vi "IRR-check-timeframe.vi"(8 "error in":errorcluster, 10 "Clk":dbl, 11 "ProcName":string) -> (0 "error out":errorcluster, 1 "ENG.CALL":cluster{"CMD":T1, "data":variant}, 2 "Report":string, 5 "Will Irrigate?":bool)   [LabVIEW 2024]
uses:
  controls/state-engine.ctl
  controls/type.eng-call.proc-insert.ctl
  controls/UiStepBuilder.ctl
  controls/type.step-builder.ctl
  io.interface.serial.vi
  build.flowToVarient.vi
  <vilib>/Utility/error.llb/Clear Errors.vi
  Polymorphics/variantCtrl.polymorphic.vi
  Polymorphics/variantCtrlStepFunction.vi
  Polymorphics/variantCtrlSetpoint.vi
  Polymorphics/variantCtrlString.vi
  proc.util.enumToStrStepVar.vi
  util.DelimitedStringFromArray.vi
  Polymorphics/variantCtrlNumber.vi
  util.DelimitedStringToArray.vi
  proc.util.validateParamExist.vi
  <vilib>/Utility/error.llb/Trim Whitespace.vi
  <vilib>/Utility/error.llb/Trim Whitespace One-Sided.vi
  globals/globals-engine.vi
  Polymorphics/variantCtrlIo.vi
  util.environment.vi
  util-address-parser.vi
  util-address-builder.vi
  util.DO.ToString.vi
  Polymorphics/io.command-builder.vi
  Polymorphics/io.command-builder.DO.vi
  Polymorphics/io.command-builder.AI.vi
  Polymorphics/io.command-builder.DI.vi
  io.frame.vi
  io.visa.vi
  io.responseValidator.vi
  Polymorphics/io.command-parser.DI.vi
  Polymorphics/io.command-parser.AI.vi
  build.elementToParamString.vi
  util.error.create.vi
  Polymorphics/variantCtrlStepPointer.vi
  Polymorphics/variantCtrlStepUserMessage.vi
  Polymorphics/variantCtrlStepPath.vi
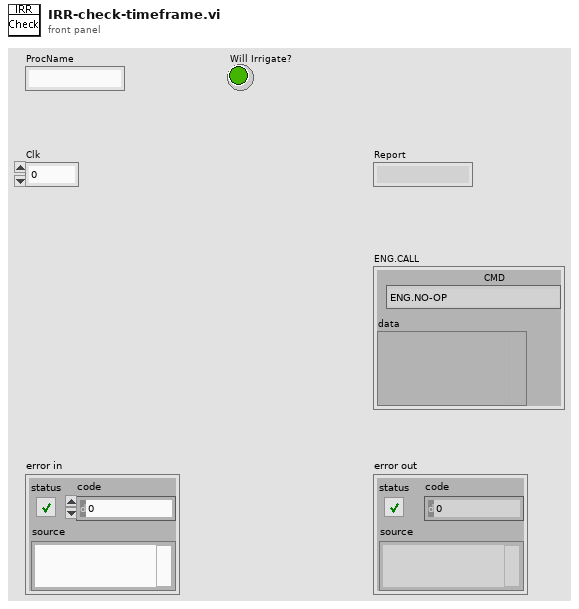
[diagram p1: front panel]
types:
  T1 = typedef "state-engine.ctl" = enum16{"ENG.NO-OP", "ENG.START", "ENG.STOP", "ENG.EXECUTE", "ENG.STATUS", "ENG.EXTERNAL-CALL", "ENG.INIT", "ENG.INIT.VARS", "ENG.INIT.SERIAL", "ENG.LOAD", "ENG.LOAD.SINGLE", "ENG.LOAD.MODULE", "ENG.LOAD.RELOAD", "ENG.LOAD.UNLOAD", "ENG.IO.LOAD", "ENG.IO.SAVE", "ENG.PROC.RELOAD-BY-NAME", "ENG.PROC.START", "ENG.PROC.STOP", "ENG.PROC.INSERT-STEPS", "ENG.PROC.ISRUNNING", "ENG.PROC.PRESET", "ENG.PROC.STATUS", "ENG.PRINT-USER-MSG", "ENG.RIO.SNAPSHOT", "ENG.RIO.AIN-SNAPSHOT-CALIB", "ENG.RIO.DOUT-BY-ADDR", "ENG.RIO.DOUT-BY-NAME", "ENG.RIO.RFS-DELAY-SET-X1", "ENG.RIO.RFS-DELAY-SET-X8", "ENG.RIO.RFS-CYCLES-SET", "ENG.RIO.RFS-CYCLES-GET", "ENG.RIO.RFS-ENABLE", "ENG.EXIT"}
  T2 = typedef "type.eng-call.proc-insert.ctl" = cluster{"ProcName":string, "instructions":variant[]}
  T3 = typedef "irr-panel.ctl" = cluster{"Day Time":cluster{"Sunset":timestamp, "Sunrise":timestamp}, "timeLimits":cluster{"Irrigation":dbl, "Nut./Water":dbl}, "Calculated Timing":cluster{"Irrigation Timeout":timestamp, "Nutrients Timeout":timestamp}, "Irr Dosing Time":cluster{"Nutrients":u16, "Water":u16, "Wash":u16}, "UV Limit ":dbl, "Dose Table":cluster{"Enable":bool, "output":string}[], "Last Iteration":timestamp, "UV Reduction Status":bool, "UV Reduction":u8}
  T4 = typedef "UiStepBuilder.ctl" = cluster{"Step Function":T5, "ParamString":string, "Step Label":string}
  T5 = typedef "type.step-builder.ctl" = enum16{"NO_OPERATION", "DELAY-JUMP", "DELAY", "JUMP", "COMPLETE", "SCHEDULER", "IRR-CHECK", "UNIT-CHECK", "UNIT-SAMPLE", "UNIT-DOSE", "LOG-REPORT", "LOG-MESSAGE", "IO-READ", "IO-READ-MANY", "IO-WRITE", "IO-COMPARE-OUT", "IO-COMPARE-IN", "PROC-START", "PROC-STOP", "PROC-LOAD", "PROC-IS-COMPLETED", "RECORD-MOVE", "GET-RH", "GET-UV", "GET-WD", "GET-WS", "OCS-CHECK", "OCS-RECORD"}
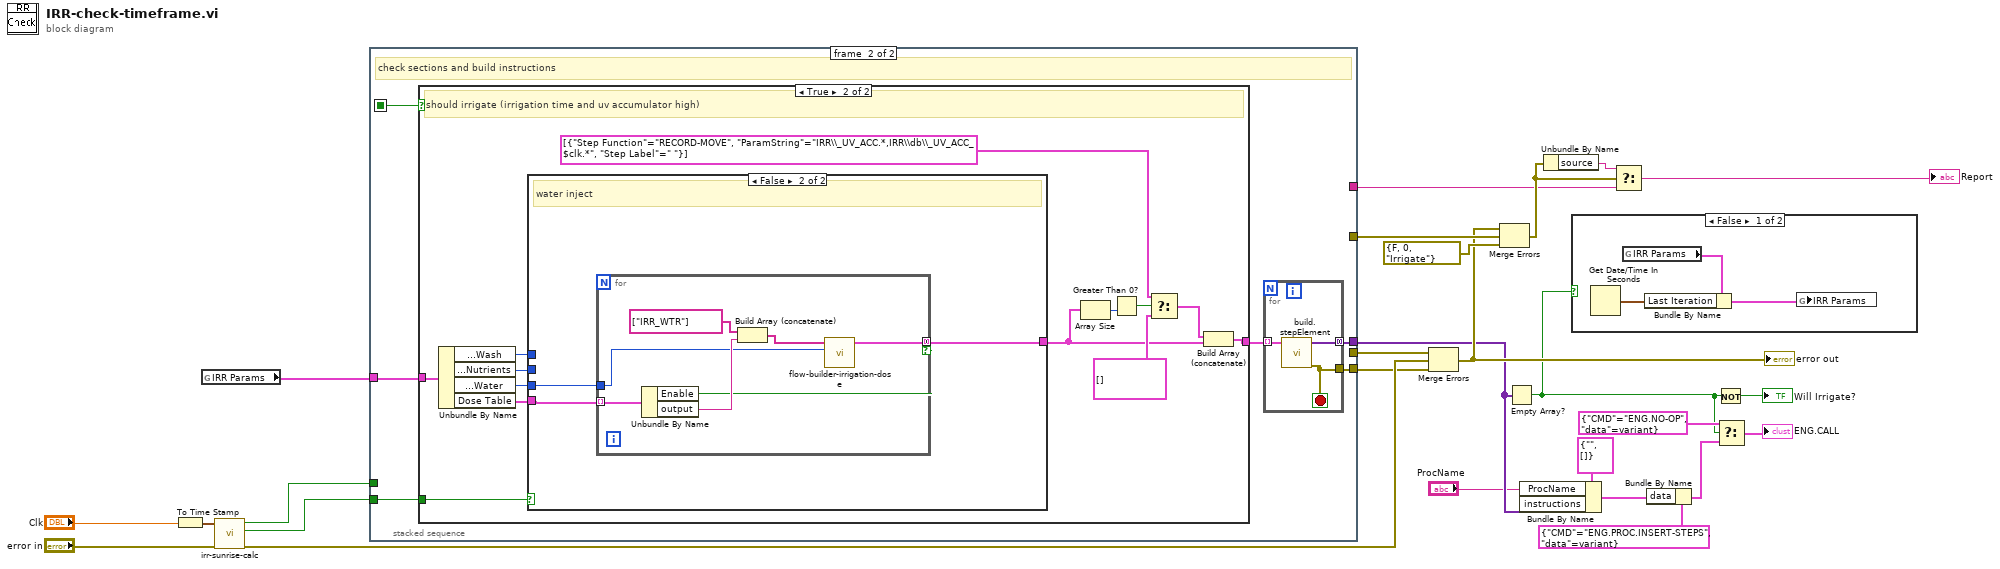
[diagram p0: block diagram]
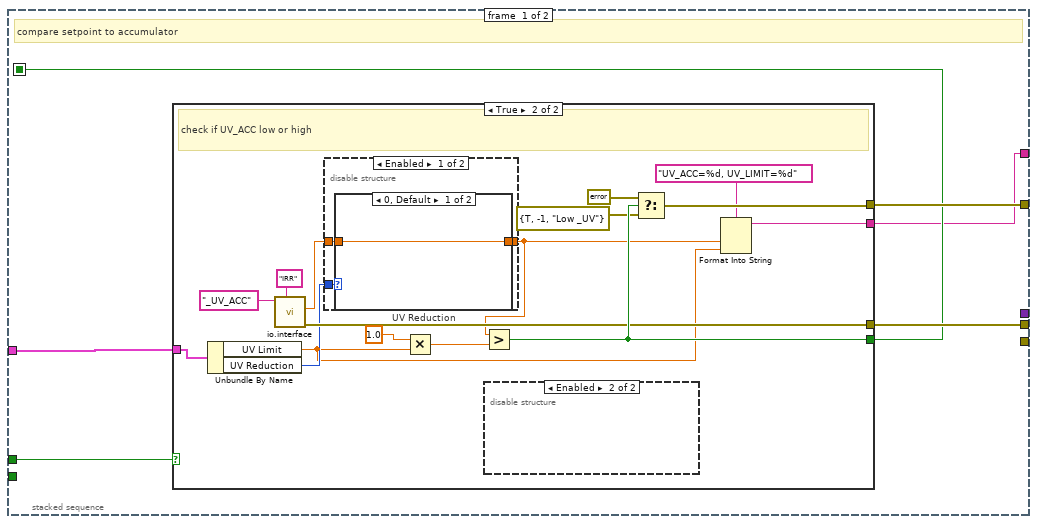
[diagram p3: hidden frame]
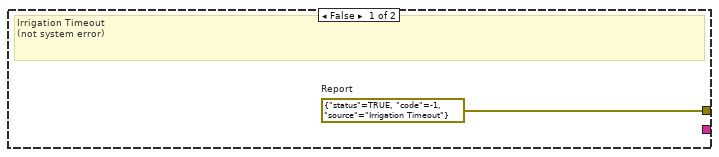
[diagram p4: hidden frame]
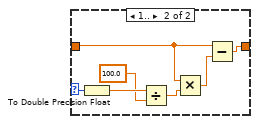
[diagram p5: hidden frame]
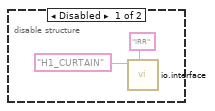
[diagram p7: hidden frame]
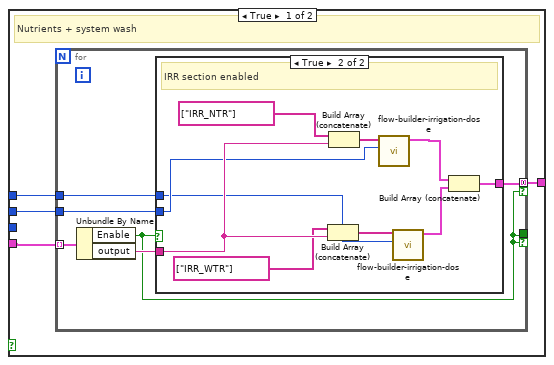
[diagram p9: hidden frame]
diagram:
  n1 = To Time Stamp(1:"Clk") -> (0:w20:timestamp)
  n2 = global read "globals-engine.vi" "IRR Params"() -> (w18:T3)
  n3 = call "irr-sunrise-calc.vi"("error in"="error in", "Time Stamp"=w20) -> ("error out"=w25:errorcluster, "(T) Nutrients (F) Water"=w16:bool, "Irrigation Time"=w17:bool)  [unwired: 6 in, 1 out]
  n4 = stacked-sequence {
    seq-local: [w28 _] -> [_ w69]
    tunnel: [w32 _] -> w24
    tunnel: [w31 _] -> w22
    tunnel: w18 -> [w30 w67]
    tunnel: w17 -> [w29 _]
    tunnel: w16 -> [_ w68]
    tunnel: [_ w65] -> w15
    tunnel: [_ w64] -> w6
    tunnel: [w27 _] -> w2
    frame #0 {
      # "compare setpoint to accumulator"
      n5 = case shown="True" w29 {
        tunnel: [_ w46] -> w31
        tunnel: [_ w49] -> w28
        tunnel: [w33 w45] -> w32
        tunnel: w30 -> [_ w43]
        tunnel: [_ w36] -> w27
        frame False {
          w33 = errorcluster {"status"=TRUE, "code"=-1, "source"="Irrigation Timeout"}  # Report
          # "Irrigation Timeout\n(not system error)"
        }
        frame True {
          # "check if UV_ACC low or high"
          n6 = Unbundle By Name(w43) -> ("UV Limit"=w38:dbl, "UV Reduction"=w40:u8)
          n7 = call "io.interface.vi"("Caller"="IRR", "IO Name in"="_UV_ACC") -> ("error out"=w46:errorcluster, "Value out"=w41:dbl)  [unwired: 4 in, 4 out]
          n8 = disable-structure shown="Enabled" {
            disable-tunnel: w41 -> [w52 w61]
            disable-tunnel: [w51 w61] -> w39
            disable-tunnel: w40 -> [w50 _]
            frame Enabled {
              n9 = case "UV Reduction" shown="0, Default" w50 {
                selector: w50 -> [_ w60]
                tunnel: w52 -> [w53 w59]
                tunnel: [w53 w57] -> w51
                frame 0, Default {
                }
                frame 1.. {
                  n10 = To Double Precision Float(number=w60) -> (double precision float=w56:dbl)
                  n11 = Divide(x=w56, y=100.0) -> (x/y=w54:dbl)
                  n12 = Multiply(x=w59, y=w54) -> (x*y=w58:dbl)
                  n13 = Subtract(x=w59, y=w58) -> (x-y=w57:dbl)
                }
              }
            }
            frame Disabled {
            }
          }
          n14 = Multiply(x=1.0, y=w38) -> (x*y=w35:dbl)
          n15 = Greater?(x=w39, y=w35) -> (0:w49:bool)
          n16 = disable-structure shown="Enabled" {
            frame Disabled {
              n17 = call "io.interface.vi"("Caller"="IRR", "IO Name in"="H1_CURTAIN") -> ()  [unwired: 4 in, 6 out]
            }
            frame Enabled {
            }
          }
          n18 = Select(t=errorcluster {"status"=FALSE, "code"=0, "source"=""}, s=w49, f=errorcluster {"status"=TRUE, "code"=-1, "source"="Low _UV"} ("error IO")) -> (s? t:f=w45:errorcluster)
          n19 = Format Into String(format string="UV_ACC=%d, UV_LIMIT=%d", w39, w38) -> (resulting string=w36:string)  [unwired: 2 in, 1 out]
        }
      }
    }
    frame #1 {
      # "check sections and build instructions"
      n20 = case shown="True" w69 {
        tunnel: w68 -> [_ w81]
        tunnel: [_ w79] -> w66
        tunnel: w67 -> [_ w80]
        frame False {
          # "should NOT irrigate (irrigation timeout or uv accumulator low)"
        }
        frame True {
          # "should irrigate (irrigation time and uv accumulator high)"
          n21 = Unbundle By Name(w80) -> ("Irr Dosing Time.Wash"=w84:u16, "Irr Dosing Time.Nutrients"=w83:u16, "Irr Dosing Time.Water"=w85:u16, "Dose Table"=w82:cluster{"Enable":bool, "output":string}[])
          n22 = case shown="False" w81 {
            tunnel: [w89 w108] -> w75
            tunnel: w82 -> [w88 w107]
            tunnel: w83 -> [w87 _]
            tunnel: w84 -> [w86 _]
            tunnel: w85 -> [_ w106]
            frame True {
              # "Nutrients + system wash"
              n23 = for {
                tunnel: [w92] -> w89 mode=concatenating if=w90
                tunnel: w88 -> [w95] mode=indexing
                tunnel: w87 -> [w94]
                tunnel: w86 -> [w93]
                tunnel: [w90] -> _ if=w90
                n24 = Unbundle By Name(w95) -> ("Enable"=w90:bool, "output"=w91:string)
                n25 = case shown="True" w90 {
                  tunnel: w94 -> [_ w101]
                  tunnel: w93 -> [_ w100]
                  tunnel: [_ w104] -> w92
                  tunnel: w91 -> [_ w103]
                  frame False {
                    # "IRR section diabled"
                  }
                  frame True {
                    # "IRR section enabled"
                    n26 = Build Array (concatenate)(string[] ["IRR_WTR"] ("OUTPUT"), w103) -> (w96:string[])
                    n27 = Build Array (concatenate)(string[] ["IRR_NTR"] ("OUTPUT"), w103) -> (w97:string[])
                    n28 = call "flow-builder-irrigation-dose.vi"("Digital Timeout"=w101, "OUTPUT(+AUX)"=w97) -> ("Flow"=w105:T4[])  [unwired: 9 in]
                    n29 = call "flow-builder-irrigation-dose.vi"("Digital Timeout"=w100, "OUTPUT(+AUX)"=w96) -> ("Flow"=w102:T4[])  [unwired: 9 in]
                    n30 = Build Array (concatenate)(w105, w102) -> (w104:T4[])
                  }
                }
              }
            }
            frame False {
              # "water inject"
              n31 = for {
                tunnel: [w114] -> w108 mode=concatenating if=w109
                tunnel: w107 -> [w115] mode=indexing
                tunnel: w106 -> [w110]
                n32 = Unbundle By Name(w115) -> ("Enable"=w109:bool, "output"=w113:string)
                n33 = Build Array (concatenate)(string[] ["IRR_WTR"] ("OUTPUT"), w113) -> (w112:string[])
                n34 = call "flow-builder-irrigation-dose.vi"("Digital Timeout"=w110, "OUTPUT(+AUX)"=w112) -> ("Flow"=w114:T4[])  [unwired: 9 in]
              }
            }
          }
          n35 = Array Size(array=w75) -> (size(s)=w74:i32)
          n36 = Greater Than 0?(x=w74) -> (x > 0?=w73:bool)
          n37 = Select(t=T4[] [{"Step Function"=enum."RECORD-MOVE", "ParamString"="IRR\\_UV_ACC.*,IRR\\db\\_UV_ACC_$clk.*", "Step Label"=" "}] ("Flow"), s=w73, f=T4[] [] ("array")) -> (s? t:f=w76:T4[])
          n38 = Build Array (concatenate)(w76, w75) -> (w79:T4[])
        }
      }
      n39 = for {
        tunnel: w66 -> [w72] mode=indexing
        tunnel: [w71] -> w65 mode=concatenating
        tunnel: [w70] -> w64
        stop <- w70 stop-if-true
        n40 = call "build.stepElement.vi"("Step in"=w72) -> ("error out"=w70:errorcluster, "steps out"=w71:variant[])  [unwired: 9 in]
      }
    }
  }
  n41 = Merge Errors(w22, w25, w6) -> (w19:errorcluster)
  "error out" <- w19
  n42 = Merge Errors(w19, w24, errorcluster {"status"=FALSE, "code"=0, "source"="Irrigate"} ("error in")) -> (w4:errorcluster)
  n43 = Empty Array?(array=w15) -> (empty?=w5:bool)
  n44 = Bundle By Name(cluster=T2 {"ProcName"="", "instructions"=[]}, "ProcName"="ProcName", "instructions"=w15) -> (w10:T2)
  n45 = Unbundle By Name(w4) -> ("source"=w3:string)
  n46 = case shown="False" w5 {
    frame False {
      n47 = Get Date/Time In Seconds() -> (seconds since 1Jan1904=w118:timestamp)
      n48 = global read "globals-engine.vi" "IRR Params"() -> (w116:T3)
      n49 = Bundle By Name(cluster=w116, "Last Iteration"=w118) -> (w117:T3)
      n50 = global write "globals-engine.vi" "IRR Params"(w117) -> ()
    }
    frame True {
    }
  }
  n51 = Select(t=w3, s=w4, f=w2) -> (s? t:f=→"Report":string)
  n52 = Bundle By Name(cluster=cluster{"CMD":T1, "data":variant} {"CMD"=enum."ENG.PROC.INSERT-STEPS", "data"=variant} ("element"), "data"=w10) -> (w9:cluster{"CMD":T1, "data":variant})
  n53 = Not(x=w5) -> (.not. x?=→"Will Irrigate?":bool)
  n54 = Select(t=cluster{"CMD":T1, "data":variant} {"CMD"=enum."ENG.NO-OP", "data"=variant} ("element"), s=w5, f=w9) -> (s? t:f=→"ENG.CALL":cluster{"CMD":T1, "data":variant})
